vi "Periodic Tasks.vi"(8 "error in":errorcluster) -> ()   [LabVIEW 2012]
doc: "This VI runs in parallel to other tasks. It can contain as many user-defined periodic loops as you need. These can carry out PID or other sorts of timed response."
uses:
  <vilib>/Rock Robotics/SystemInterfaces/Utilities/FPGA_UtilitiesLED Source.ctl
  <vilib>/Rock Robotics/SystemInterfaces/Utilities/FPGA_UtilitiesLED State.ctl
  <vilib>/Rock Robotics/WPI/Compressor/WPI_CompressorGetSetRefNum.vi
  Robot Global Data.vi
  <vilib>/Rock Robotics/WPI/Joystick/WPI_JoystickGetSetRefNum.vi
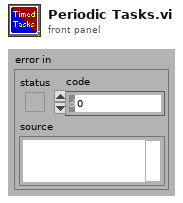
[diagram p1: front panel]
types:
  T1 = typedef "FPGA_UtilitiesLED State.ctl" = enum16{"Off", "On", "Toggle"}
  T2 = typedef "FPGA_UtilitiesLED Source.ctl" = enum16{"User LED", "FPGA LED"}
  T3 = typedef "WPI_CompressorDevRef.ctl" = cluster{"DevStatus":errorcluster, "DigitalInputDevRef":T4, "RelayDevRef":T7}
  T4 = typedef "WPI_DigitalInputDevRef.ctl" = cluster{"DevStatus":errorcluster, "DIO Channel":T5, "Digital Module":T6}
  T5 = typedef "FPGA_DIOChannel.ctl" = enum8{"DIO 1", "DIO 2", "DIO 3", "DIO 4", "DIO 5", "DIO 6", "DIO 7", "DIO 8", "DIO 9", "DIO 10", "DIO 11", "DIO 12", "DIO 13", "DIO 14", "Invalid"}
  T6 = typedef "FPGA_TypedefDigitalModule.ctl" = enum16{"Digital Module 1", "Digital Module 2"}
  T7 = typedef "WPI_RelayDevRef.ctl" = cluster{"DevStatus":errorcluster, "Relay Channel":T8, "Digital Module":T6, "Relay Direction":T9}
  T8 = typedef "FPGA_DIORelayChannel.ctl" = enum8{"Relay 1", "Relay 2", "Relay 3", "Relay 4", "Relay 5", "Relay 6", "Relay 7", "Relay 8", "Invalid"}
  T9 = typedef "WPI_RelayDirection.ctl" = enum16{"Both directions", "Forward only", "Reverse only"}
  T10 = typedef "WPI_JoystickDevRef.ctl" = cluster{"Device":T11}
  T11 = typedef "WPI_JoystickDeviceEnum.ctl" = enum16{"USB 1", "USB 2", "USB 3", "USB 4", "Kinect 1", "Kinect 2"}
  T12 = typedef "WPI_JoystickButtonState.ctl" = cluster{"Button 1":bool, "Button 2":bool, "Button 3":bool, "Button 4":bool, "Button 5":bool, "Button 6":bool, "Button 7":bool, "Button 8":bool, "Button 9":bool, "Button 10":bool, "Button 11":bool, "Button 12":bool}
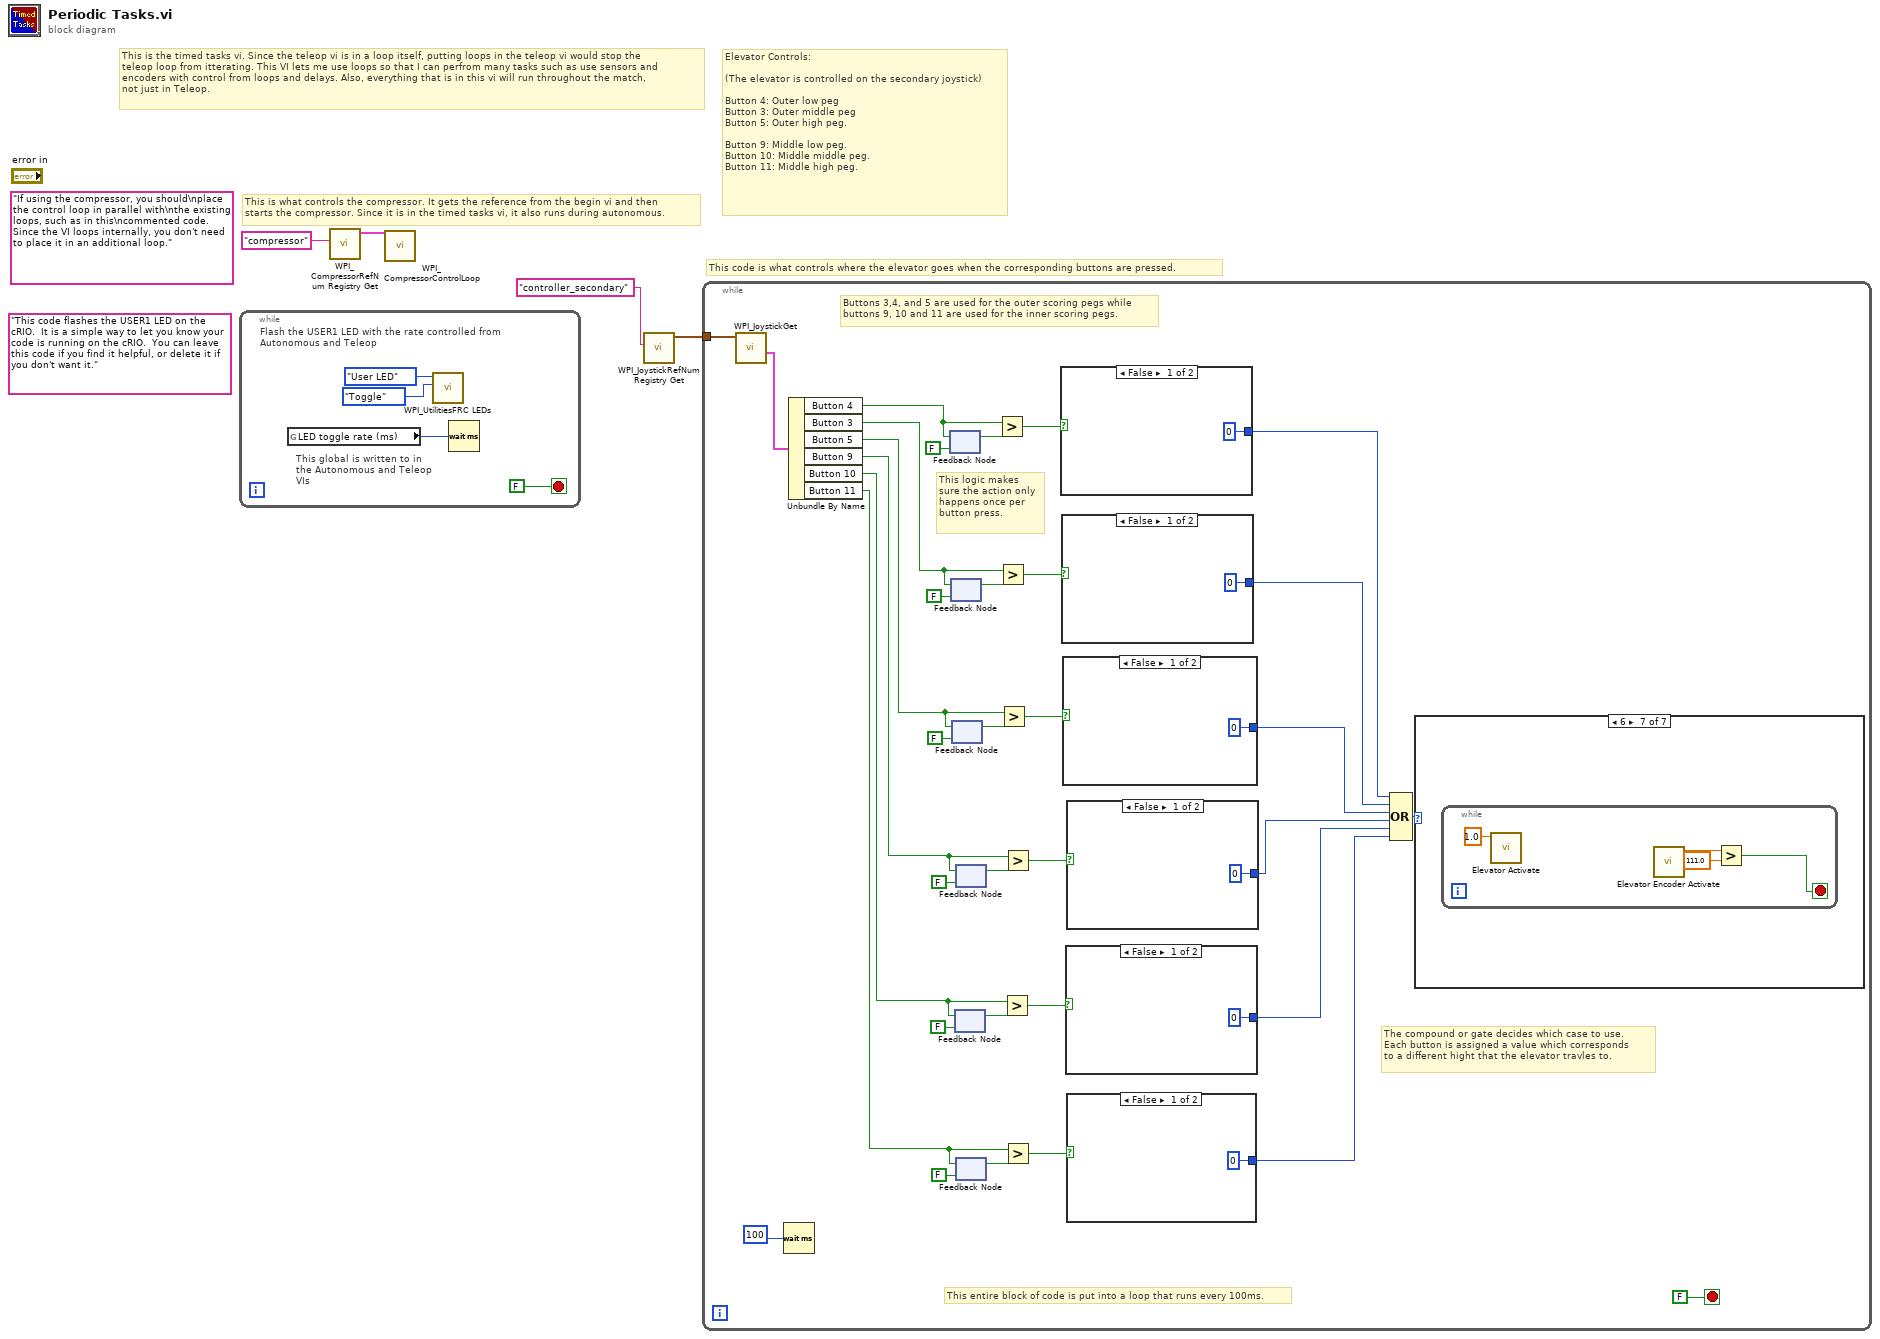
[diagram p0: block diagram]
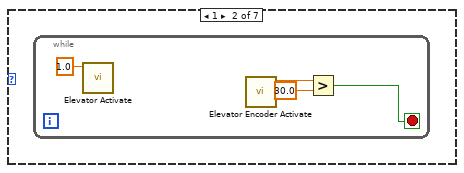
[diagram p3: hidden frame]
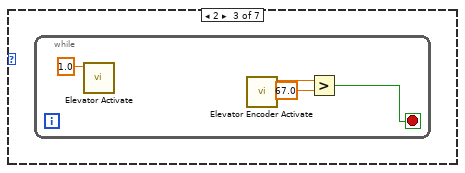
[diagram p4: hidden frame]
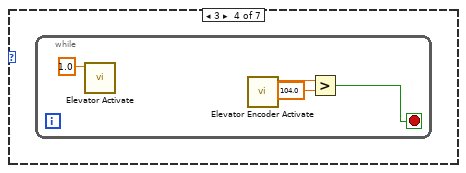
[diagram p5: hidden frame]
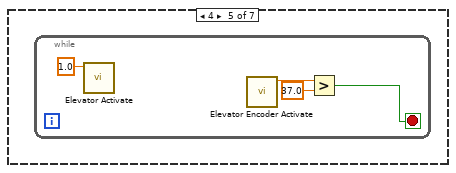
[diagram p6: hidden frame]
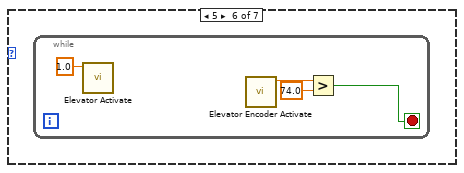
[diagram p7: hidden frame]
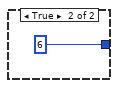
[diagram p8: hidden frame]
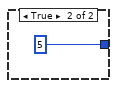
[diagram p9: hidden frame]
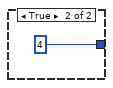
[diagram p10: hidden frame]
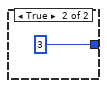
[diagram p11: hidden frame]
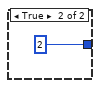
[diagram p12: hidden frame]
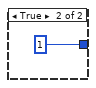
[diagram p13: hidden frame]
diagram:
  (unwired) "If using the compressor, you should\nplace the control loop in parallel with\nthe existing loops, such as in this\ncommented code. Since the VI loops internally, you don't need to place it in an additional loop."
  (unwired) "This code flashes the USER1 LED on the cRIO.  It is a simple way to let you know your code is running on the cRIO.  You can leave this code if you find it helpful, or delete it if you don't want it."
  # "Elevator Controls: \n\n(The elevator is controlled on the secondary joystick) \n\nButton 4: Outer low peg \nButton 3: Outer middle peg \nButton 5: Outer high peg. \n\nButton 9: Middle low peg. \nButton 10: Middle middle peg. \nButton 11: Middle high peg."
  # "This code is what controls where the elevator goes when the corresponding buttons are pressed."
  # "This is what controls the compressor. It gets the reference from the begin vi and then \nstarts the compressor. Since it is in the timed tasks vi, it also runs during autonomous."
  # "This is the timed tasks vi. Since the teleop vi is in a loop itself, putting loops in the teleop vi would stop the \nteleop loop from itterating. This VI lets me use loops so that I can perfrom many tasks such as use sensors and \nencoders with control from loops and delays. Also, everything that is in this vi will run throughout the match, \nnot just in Teleop."
  n1 = while {
    stop <- FALSE stop-if-true
    # "This global is written to in the Autonomous and Teleop VIs"
    # "Flash the USER1 LED with the rate controlled from Autonomous and Teleop"
    n2 = global read "Robot Global Data.vi" "LED toggle rate (ms)"() -> (w5:u32)
    n3 = call <vilib>:"WPI_UtilitiesFRC LEDs.vi"("State"=FPGA_UtilitiesLED_State."Toggle", "LED Type"=FPGA_UtilitiesLED_Source."User LED") -> ()  [unwired: 1 in, 9 out]
    n4 = Wait (ms)(milliseconds to wait=w5) -> ()  [unwired: 1 out]
  }
  n5 = call <vilib>:"WPI_CompressorRefNum Registry Get.vi"("refnum name"="compressor") -> ("CompressorDevRef"=w4:T3)  [unwired: 9 in, 1 out]
  n6 = call <vilib>:"WPI_CompressorControlLoop.vi"("CompressorDevRef"=w4) -> ()  [unwired: 11 in]
  n7 = call <vilib>:"WPI_JoystickRefNum Registry Get.vi"("refnum name"="controller_secondary") -> ("JoystickDevRef"=w1:T10)  [unwired: 9 in, 1 out]
  n8 = while {
    tunnel: w1 -> [w43]
    stop <- FALSE stop-if-true
    # "This entire block of code is put into a loop that runs every 100ms."
    # "The compound or gate decides which case to use. \nEach button is assigned a value which corresponds \nto a different hight that the elevator travles to."
    # "This logic makes \nsure the action only\nhappens once per \nbutton press."
    # "Buttons 3,4, and 5 are used for the outer scoring pegs while \nbuttons 9, 10 and 11 are used for the inner scoring pegs."
    n9 = call <vilib>:"WPI_JoystickGet.vi"("JoystickDevRef"=w43) -> ("Buttons"=w40:T12)  [unwired: 4 in, 2 out]
    n10 = Wait (ms)(milliseconds to wait=u32 100) -> ()  [unwired: 1 out]
    n11 = Unbundle By Name(w40) -> ("Button 4"=w33:bool, "Button 3"=w32:bool, "Button 5"=w28:bool, "Button 9"=w24:bool, "Button 10"=w20:bool, "Button 11"=w16:bool)
    n12 = feedback-in #1(w33) -> ()
    n13 = feedback #1(FALSE ("Button 2")) -> (w39:bool)
    n14 = feedback #2(FALSE ("Button 2")) -> (w34:bool)
    n15 = feedback-in #2(w32) -> ()
    n16 = feedback #3(FALSE ("Button 2")) -> (w29:bool)
    n17 = feedback-in #3(w28) -> ()
    n18 = feedback #4(FALSE ("Button 2")) -> (w21:bool)
    n19 = feedback-in #4(w20) -> ()
    n20 = feedback #5(FALSE ("Button 2")) -> (w27:bool)
    n21 = feedback-in #5(w24) -> ()
    n22 = feedback #6(FALSE ("Button 2")) -> (w19:bool)
    n23 = feedback-in #6(w16) -> ()
    n24 = Greater?(x=w33, y=w39) -> (0:w37:bool)
    n25 = Greater?(x=w32, y=w34) -> (0:w36:bool)
    n26 = Greater?(x=w28, y=w29) -> (0:w31:bool)
    n27 = Greater?(x=w20, y=w21) -> (0:w23:bool)
    n28 = Greater?(x=w24, y=w27) -> (0:w25:bool)
    n29 = Greater?(x=w16, y=w19) -> (0:w17:bool)
    n30 = case shown="False" w37 {
      tunnel: [0 1] -> w15
      frame False {
      }
      frame True {
      }
    }
    n31 = case shown="False" w36 {
      tunnel: [0 2] -> w14
      frame False {
      }
      frame True {
      }
    }
    n32 = case shown="False" w31 {
      tunnel: [0 3] -> w13
      frame False {
      }
      frame True {
      }
    }
    n33 = case shown="False" w23 {
      tunnel: [0 5] -> w11
      frame False {
      }
      frame True {
      }
    }
    n34 = case shown="False" w25 {
      tunnel: [0 4] -> w12
      frame False {
      }
      frame True {
      }
    }
    n35 = case shown="False" w17 {
      tunnel: [0 6] -> w10
      frame False {
      }
      frame True {
      }
    }
    n36 = Compound Arithmetic op=OR(w15, w14, w13, w12, w11, w10) -> (w9:i32)
    n37 = case shown="6" w9 {
      frame 0, Default {
        # "DOES NOTHING"
      }
      frame 1 {
        n38 = while {
          stop <- w45 stop-if-true
          n39 = call "Elevator Activate.vi"("Elevator Output"=1.0) -> ()  [unwired: 11 in]
          n40 = call "Elevator Encoder Activate.vi"() -> ("Distance"=w46:dbl)  [unwired: 11 in]
          n41 = Greater?(x=w46, y=30.0) -> (0:w45:bool)
        }
      }
      frame 2 {
        n42 = while {
          stop <- w49 stop-if-true
          n43 = call "Elevator Activate.vi"("Elevator Output"=1.0) -> ()  [unwired: 11 in]
          n44 = call "Elevator Encoder Activate.vi"() -> ("Distance"=w50:dbl)  [unwired: 11 in]
          n45 = Greater?(x=w50, y=67.0) -> (0:w49:bool)
        }
      }
      frame 3 {
        n46 = while {
          stop <- w53 stop-if-true
          n47 = call "Elevator Activate.vi"("Elevator Output"=1.0) -> ()  [unwired: 11 in]
          n48 = call "Elevator Encoder Activate.vi"() -> ("Distance"=w54:dbl)  [unwired: 11 in]
          n49 = Greater?(x=w54, y=104.0) -> (0:w53:bool)
        }
      }
      frame 4 {
        n50 = while {
          stop <- w57 stop-if-true
          n51 = call "Elevator Activate.vi"("Elevator Output"=1.0) -> ()  [unwired: 11 in]
          n52 = call "Elevator Encoder Activate.vi"() -> ("Distance"=w58:dbl)  [unwired: 11 in]
          n53 = Greater?(x=w58, y=37.0) -> (0:w57:bool)
        }
      }
      frame 5 {
        n54 = while {
          stop <- w61 stop-if-true
          n55 = call "Elevator Activate.vi"("Elevator Output"=1.0) -> ()  [unwired: 11 in]
          n56 = call "Elevator Encoder Activate.vi"() -> ("Distance"=w62:dbl)  [unwired: 11 in]
          n57 = Greater?(x=w62, y=74.0) -> (0:w61:bool)
        }
      }
      frame 6 {
        n58 = while {
          stop <- w65 stop-if-true
          n59 = call "Elevator Activate.vi"("Elevator Output"=1.0) -> ()  [unwired: 11 in]
          n60 = call "Elevator Encoder Activate.vi"() -> ("Distance"=w66:dbl)  [unwired: 11 in]
          n61 = Greater?(x=w66, y=111.0) -> (0:w65:bool)
        }
      }
    }
  }
